vi "Start Triggers Time Core.vi"(0 "rx.trigger select":T4=enum."Immediate", 1 "time.resources":T3, 5 "rx.trigger enable":bool, 7 "rx.software trigger":bool, 9 "rx.stream enable":bool, 11 "tx.trigger select":T4=enum."Immediate", 12 "tx.trigger enable":bool, 13 "tx.software trigger":bool, 14 "tx.stream enable":bool) -> (4 "rx.start trigger":bool, 6 "tx.start trigger":bool)   [LabVIEW 2016]
uses:
  HOST/29x5/SubVIs/Start Trigger.ctl
  <instrlib>/niUsrpRio/Time/v1/FPGA/Private/Time Resources.ctl
  <instrlib>/niUsrpRio/Time/v1/FPGA/Private/Future Event Resources.ctl
  <instrlib>/niUsrpRio/Time/v1/FPGA/niUsrpRio Time v1 FPGA.lvlib
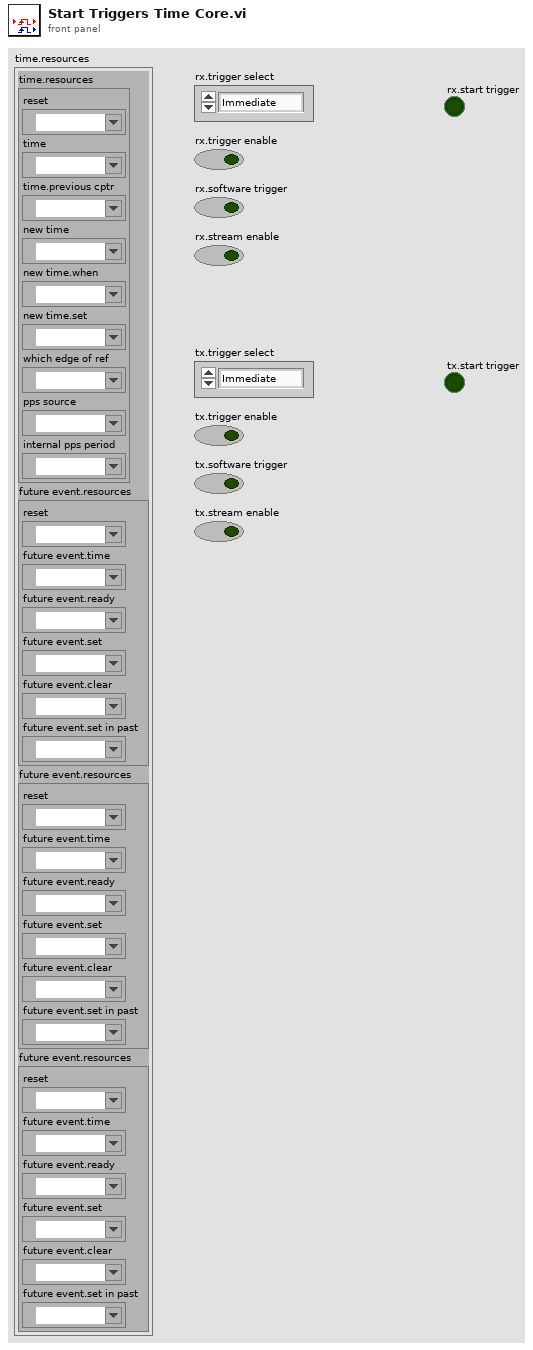
[diagram p1: front panel]
types:
  T1 = typedef "niUsrpRio Time v1 FPGA.lvlib/Time Resources.ctl" = cluster{"reset":refnum<k21>, "time":refnum<k21>, "time.previous cptr":refnum<k21>, "new time":refnum<k21>, "new time.when":refnum<k21>, "new time.set":refnum<k21>, "which edge of ref":refnum<k21>, "pps source":refnum<k21>, "internal pps period":refnum<k21>}
  T2 = typedef "niUsrpRio Time v1 FPGA.lvlib/Future Event Resources.ctl" = cluster{"reset":refnum<k21>, "future event.time":refnum<k21>, "future event.ready":refnum<k21>, "future event.set":refnum<k21>, "future event.clear":refnum<k21>, "future event.set in past":refnum<k21>}
  T3 = cluster{"time.resources":T1, "future event.resources":T2, "future event.resources":T2, "future event.resources":T2}
  T4 = typedef "Start Trigger.ctl" = enum8{"Software", "Digital Edge", "Rx Start Trigger", "Tx Start Trigger", "Immediate", "Future Time Event"}
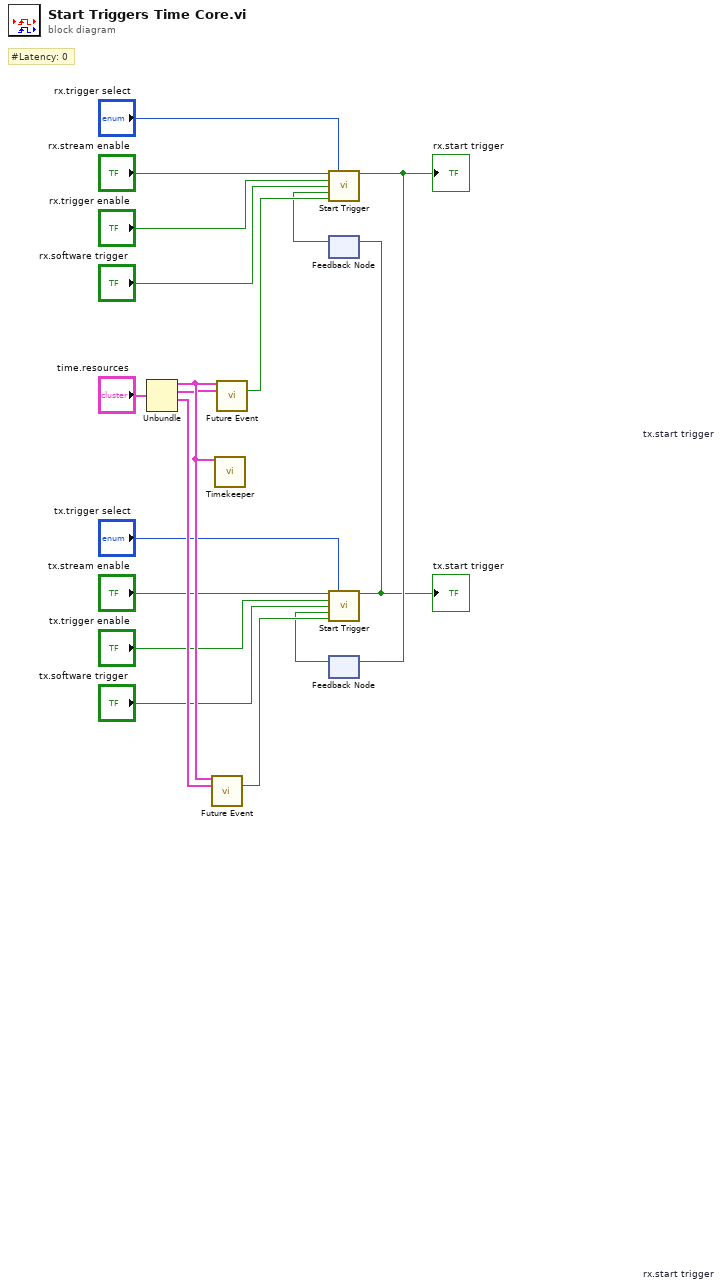
[diagram p0: block diagram]
diagram:
  # "#Latency: 0"
  n1 = Unbundle("time.resources") -> ("time.resources"=w18:T1, "future event.resources"=w4:T2, "future event.resources"=w17:T2)  [unwired: 1 out]
  n2 = call <instrlib>:"Future Event.vi"("time.resources"=w18, "future event.resources"=w17) -> ("event.occurred"=w10:bool)  [unwired: 12 in, 1 out]
  n3 = call <instrlib>:"Timekeeper.vi"("time.resources"=w18) -> ()  [unwired: 13 in, 2 out]
  n4 = call <instrlib>:"Future Event.vi"("time.resources"=w18, "future event.resources"=w4) -> ("event.occurred"=w9:bool)  [unwired: 12 in, 1 out]
  n5 = feedback #1 "tx.start trigger"() -> (w5:bool)  [unwired: 1 in]
  n6 = call "Start Trigger.vi"("stream enable"="rx.stream enable", "trigger select"="rx.trigger select", "trigger enable"="rx.trigger enable", "software trigger"="rx.software trigger", "other start trigger"=w5, "event occurred"=w9) -> ("start trigger"=w12:bool)  [unwired: 9 in]
  "rx.start trigger" <- w12
  n7 = feedback-in #2(w12) -> ()
  n8 = feedback #2 "rx.start trigger"() -> (w6:bool)  [unwired: 1 in]
  n9 = call "Start Trigger.vi"("stream enable"="tx.stream enable", "trigger select"="tx.trigger select", "trigger enable"="tx.trigger enable", "software trigger"="tx.software trigger", "other start trigger"=w6, "event occurred"=w10) -> ("start trigger"=w11:bool)  [unwired: 9 in]
  "tx.start trigger" <- w11
  n10 = feedback-in #1(w11) -> ()
